vi "Run Bfr Rx - Check Valid Buffer.vi"(8 "error in (no error)":errorcluster, 11 "Rx Loop Data in":T1 {"Data Buffer" format="%016x"}) -> (0 "error out":errorcluster, 2 "Allow Rx?":bool, 3 "Rx Loop Data out":T1 {"Data Buffer" format="%016x"})   [LabVIEW 2016, in "UDP-Custom-Device Engine.lvlib"]
uses:
  UDP-Custom-Device Engine.lvlib
  Types/Engine - Buffered Rx Loop Data.ctl
  Shared/Types/Shared - Header Details.ctl
  Shared/Types/Shared - Buffered.PacketInfo.ctl
  Shared/Types/Shared - Pointer Encoding.ctl
  <vilib>/NI/NIVS Inline Async API/_Data Access Engine/Data Access Engine/Types/Read.DVR.ctl
  <vilib>/NI/NIVS Inline Async API/_Data Access Engine/Access Type Classes/Read/Read.lvclass
  <vilib>/NI/NIVS Inline Async API/_Data Access Engine/Data Access Engine/Types/Write.DVR.ctl
  <vilib>/NI/NIVS Inline Async API/_Data Access Engine/Access Type Classes/Write/Write.lvclass
  Shared/Types/Shared - Duplex Settings.ctl
  <vilib>/NI/NIVS Inline Async API/_Data Access Engine/Access Type Classes/Read/Read.lvclass/Read.ctl
  <vilib>/NI/NIVS Inline Async API/_Data Access Engine/Data Access Engine/Methods/Read.Data.vi
  <vilib>/NI/NIVS Inline Async API/_Data Access Engine/Access Type Classes/Read/Read.ProcessData.vi
  <vilib>/NI/NIVS Inline Async API/_Data Access Engine/Data Access Engine/Data Access Engine.lvclass
  Shared/UDP-Custom-Device Shared.lvlib
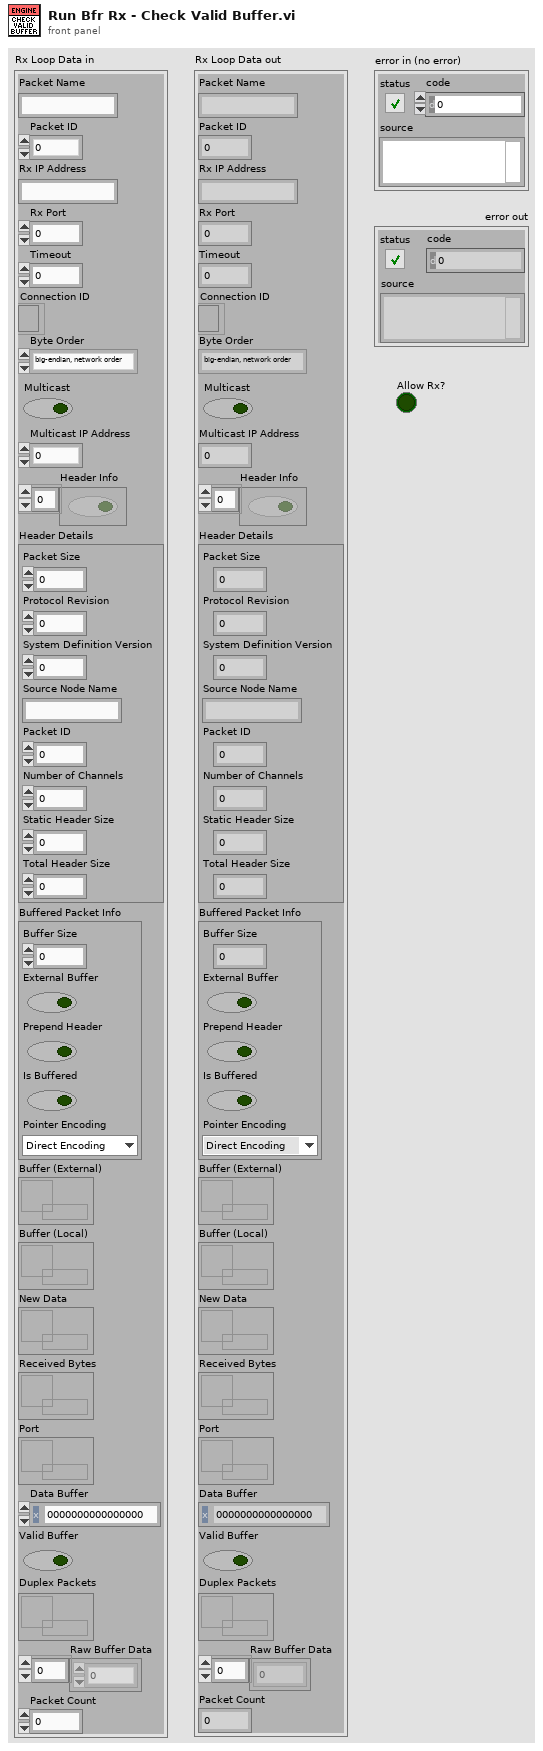
[diagram p1: front panel]
types:
  T1 = typedef "UDP-Custom-Device Engine.lvlib/Engine - Buffered Rx Loop Data.ctl" = cluster{"Packet Name":string, "Packet ID":i32, "Rx IP Address":string, "Rx Port":i32, "Timeout":i32, "Connection ID":refnum<k16>, "Byte Order":enum16{"big-endian, network order", "native, host order", "little-endian"}, "Multicast":bool, "Multicast IP Address":u32, "Header Info":bool[], "Header Details":T2, "Buffered Packet Info":T3, "Buffer (External)":T5, "Buffer (Local)":T6, "New Data":T6, "Received Bytes":T6, "Port":T6, "Data Buffer":u64, "Valid Buffer":bool, "Duplex Packets":refnum<data-value>, "Raw Buffer Data":u8[], "Packet Count":dbl}
  T2 = typedef "UDP-Custom-Device Shared.lvlib/Shared - Header Details.ctl" = cluster{"Packet Size":u16, "Protocol Revision":u8, "System Definition Version":u64, "Source Node Name":string, "Packet ID":u32, "Number of Channels":u32, "Static Header Size":u16, "Total Header Size":u16}
  T3 = typedef "UDP-Custom-Device Shared.lvlib/Shared - Buffered.PacketInfo.ctl" = cluster{"Buffer Size":i32, "External Buffer":bool, "Prepend Header":bool, "Is Buffered":bool, "Pointer Encoding":T4}
  T4 = typedef "UDP-Custom-Device Shared.lvlib/Shared - Pointer Encoding.ctl" = enum16{"Direct Encoding", "Conversion Encoding"}
  T5 = typedef "Data Access Engine.lvlib/Data Access Engine.lvclass/Read.DVR.ctl" = refnum<data-value>
  T6 = typedef "Data Access Engine.lvlib/Data Access Engine.lvclass/Write.DVR.ctl" = refnum<data-value>
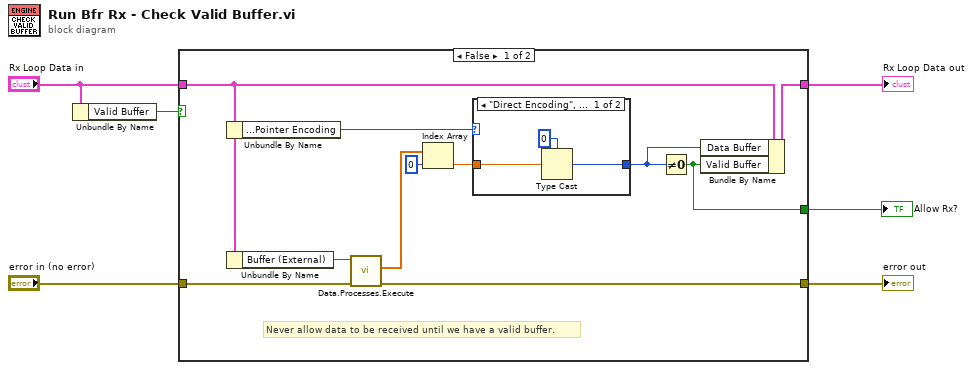
[diagram p0: block diagram]
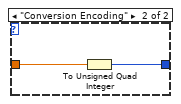
[diagram p2: hidden frame]
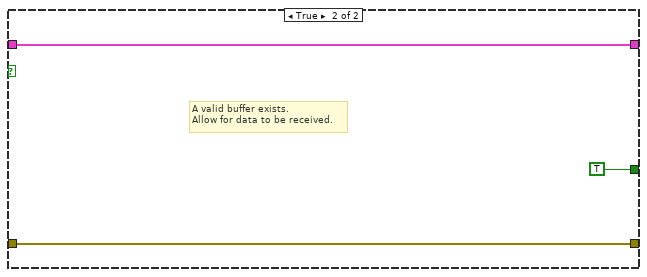
[diagram p3: hidden frame]
diagram:
  n1 = Unbundle By Name("Rx Loop Data in") -> ("Valid Buffer"=w5:bool)
  n2 = case shown="False" w5 {
    tunnel: "error in (no error)" -> [w12 w24]
    tunnel: [w14 w25] -> w3
    tunnel: "Rx Loop Data in" -> [w10 w25]
    tunnel: [w13 w24] -> w2
    tunnel: [w11 TRUE] -> w1
    frame False {
      # "Never allow data to be received until we have a valid buffer."
      n3 = Unbundle By Name(w10) -> ("Buffered Packet Info.Pointer Encoding"=w7:T4)
      n4 = Unbundle By Name(w10) -> ("Buffer (External)"=w17:T5)
      n5 = call-poly <vilib>:"Data.Processes.Execute.vi"("error in (no error)"=w12, "Ref"=w17) -> ("error out"=w13:errorcluster, "Values"=w16:dbl[])  [unwired: 7 in, 1 out]
      n6 = Index Array(array=w16, index=0) -> (element=w8:dbl)
      n7 = case shown="\"Direct Encoding\", Default" w7 {
        tunnel: w8 -> [w20 w22]
        tunnel: [w19 w21] -> w9
        frame "Direct Encoding", Default {
          n8 = Type Cast(type=u64 0, x=w20) -> (*(type *) &x=w19:u64)
        }
        frame "Conversion Encoding" {
          n9 = To Unsigned Quad Integer(1:w22) -> (0:w21:u64)
        }
      }
      n10 = Not Equal To 0?(x=w9) -> (x != 0?=w11:bool)
      n11 = Bundle By Name(cluster=w10, "Data Buffer"=w9, "Valid Buffer"=w11) -> (w14:T1)
    }
    frame True {
      # "A valid buffer exists.\nAllow for data to be received."
    }
  }
  "Rx Loop Data out" <- w3
  "error out" <- w2
  "Allow Rx?" <- w1
